vi "Accessory ID.vi"(8 "error in":errorcluster, 10 "Channel":i32(ring) items=["Input Channel 1", "Input Channel 2", "Input Channel 3", "Input Channel 4"], 11 "Instrument Handle In":i32) -> (0 "error out":errorcluster, 2 "ID String":string caption="ID", 3 "Instrument Handle Out":i32)   [LabVIEW 8.6, in "ZTScopeM.lvlib"]
doc: "Query the channel's accessory identification information"
uses:
  ZTScopeM.lvlib
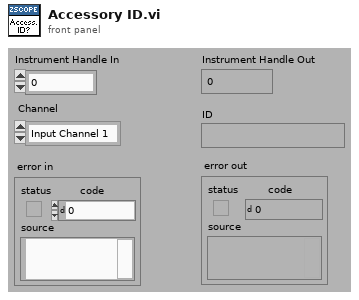
[diagram p1: front panel]
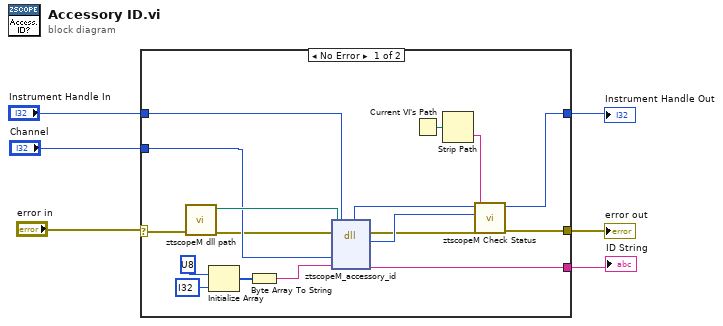
[diagram p0: block diagram]
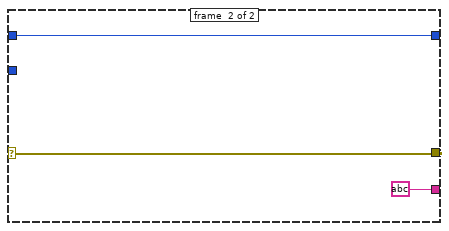
[diagram p2: hidden frame]
diagram:
  n1 = case shown="No Error" "error in" {
    selector: "error in" -> [w12 w26]
    tunnel: [w18 w26] -> w3
    tunnel: "Instrument Handle In" -> [w23 w25]
    tunnel: [w17 w25] -> w5
    tunnel: "Channel" -> [w10 _]
    tunnel: [w7 string ?] -> w1
    frame #0 {
      n2 = call "ztscopeM dll path.vi"("error in (no error)"=w12) -> ("error out"=w9:errorcluster, "<instrument>.dll path"=w11:path)  [unwired: 9 in]
      n3 = Initialize Array(u8 ?, i32 ? ("dimension size")) -> (w15:u8[])
      n4 = Byte Array To String(unsigned byte array=w15) -> (string=w13:string)
      n5 = dll-call lib="C:/Program Files (x86)/National Instruments/LabVIEW 2013/instr.lib/ztscopem/ztscopeM.dll" fn="ztscopeM_accessory_id"(path in=w11, error in=w9, "instrumentHandle"=w23, "channel"=w10, "ID"=w13) -> (error out=w8:errorcluster, w19:i32, "instrumentHandle"=w20:i32, "ID"=w7:string)  [unwired: 2 in, 1 out]
      n6 = Current VI's Path() -> (path=w22:path)
      n7 = Strip Path(path=w22) -> (name=w21:string)  [unwired: 1 out]
      n8 = call "ztscopeM Check Status.vi"("error in"=w8, "name of VI"=w21, "status (return code)"=w19, "instrument handle in"=w20) -> ("error out"=w18:errorcluster, "instrument handle out"=w17:i32)  [unwired: 2 in]
    }
    frame #1 {
    }
  }
  "Instrument Handle Out" <- w5
  "error out" <- w3
  "ID String" <- w1
